vi "IDN.vi"(2 "error in (no error)":errorcluster, 3 "VISA resource name":refnum<visa-resource-name>) -> (0 "error out":errorcluster, 1 "IDN":string)   [LabVIEW 2010]
uses:
  <vilib>/Instr/_visa.llb/VISA Configure Serial Port (Instr).vi
panel:
  out "Number of byte":u32
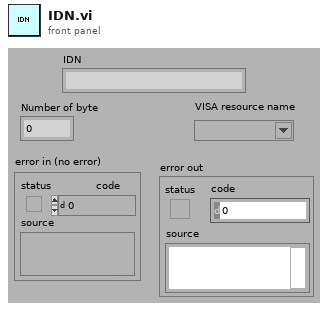
[diagram p1: front panel]
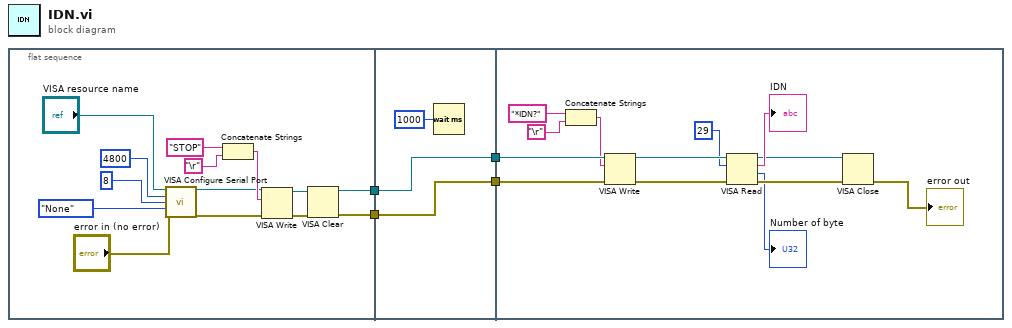
[diagram p0: block diagram]
diagram:
  n1 = flat-sequence {
    tunnel: [w5] -> w2
    tunnel: [w6] -> w1
    tunnel: [w21] -> w4
    tunnel: [w20] -> w3
    tunnel: w2 -> [w20]
    tunnel: w1 -> [w21]
    tunnel: w4 -> [w27]
    tunnel: w3 -> [w26]
    frame #0 {
      n2 = call-poly "VISA Configure Serial Port"("VISA resource name"="VISA resource name", "baud rate (9600)"=u32 4800, "data bits (8)"=u16 8, "parity (0:none)"=enum16{"None", "Odd", "Even", "Mark", "Space"}."None", "error in (no error)"="error in (no error)") -> ("VISA resource name out"=w10:refnum<visa-resource-name>, "error out"=w9:errorcluster)  [unwired: 9 in]
      n3 = Concatenate Strings("STOP" ("string"), "\r") -> (w13:string)
      n4 = VISA Write(VISA resource name=w10, write buffer=w13, error in (no error)=w9) -> (VISA resource name out=w7:refnum<visa-resource-name>, error out=w8:errorcluster)  [unwired: 1 out]
      n5 = VISA Clear(VISA resource name=w7, error in (no error)=w8) -> (VISA resource name out=w6:refnum<visa-resource-name>, error out=w5:errorcluster)
    }
    frame #1 {
      n6 = Wait (ms)(milliseconds to wait=u32 1000) -> ()  [unwired: 1 out]
    }
    frame #2 {
      n7 = Concatenate Strings("*IDN?" ("string"), "\r") -> (w24:string)
      n8 = VISA Write(VISA resource name=w27, write buffer=w24, error in (no error)=w26) -> (VISA resource name out=w33:refnum<visa-resource-name>, error out=w34:errorcluster)  [unwired: 1 out]
      n9 = VISA Read(VISA resource name=w33, byte count=u32 29, error in (no error)=w34) -> (VISA resource name out=w29:refnum<visa-resource-name>, read buffer=→"IDN":string, return count=→"Number of byte":u32, error out=w30:errorcluster)
      n10 = VISA Close(VISA resource name=w29, error in (no error)=w30) -> (error out=→"error out":errorcluster)
    }
  }
